vi "DOE Agilent Setup.vi"(8 "error in (no error)":errorcluster, 11 "Test Fixture Hardware":T1={"Power "={"Yokogawa"={"WT210"={"Sample Rate (1: 0.25s)"=1, "A Range (12: 20A)"=11, "V Range (6: 600V)"=4, "Power VISA Yokogawa WT210"=""}, "WT500"={"Power VISA Yokogawa WT500"="", "V Range (8: 1000V)"=6, "I Range (7: 40A)"=7, "Update Rate (3: 500ms)"=2}, "WT310_2"={"Sample Rate (1: 0.25s)"=1, "A Range (12: 20A)"=11, "V Range (6: 600V)"=4, "Power VISA Yokogawa WT310_2"=""}, "WT310_3"={"Sample Rate (1: 0.25s)"=1, "A Range (12: 20A)"=11, "V Range (6: 600V)"=4, "Power VISA Yokogawa WT310_3"=""}}, "Aplus"={"Aplus IP Address"="192.168.1.101", "Remote Port"=502, "Instrument"="APLUS", "Instr Driver Revision"="1.03.0053"}, "Power Limits"={"Crest Factor"={"Upper Limit"=1.49, "Lower Limit"=1.34}, "Harmonic Content"={"Uthd"=2.0}, "Voltage"={"% Error"=2.0}, "Stability"={"<1 Watt "={"Wattage"=1.0, "Slope (mW/H)"=10.0}, ">1 Watt"={"1%Power/Hour"=1.0}}}, "Nominal Voltage"=120, "Time Limit (s)"=10800.0, "Power Variation Limit (%)"=50.0, "Power Supply"={"Chroma 61605"="CHROMA", "Use Chroma?"=FALSE}}, "Weight Scale"={"Com Options"={"IND560Scale VISA"="MW100", "IP Address"="", "Remote Port"=502, "Setra Scale VISA"="MW100", "GSE 350"="GSE350"}, "Select Scale"=""}, "Flow Rates"={"Laurel Cold IP Address"="", "Laurel Hot IP Address"="", "Hot Water Laurel VISA"="LaurelMeter_Hot", "Cold Water Laurel VISA"="LaurelMeter_Cold", "Remote Port"=0, "Laurel Communication Type"="", "Meters To Collect (Hot Cold)"="", "HOT Laurel Reference"=refnum, "COLD Laurel Reference"=refnum, "Modbus Hot Ref"=refnum}, "Analog Data"={"Agilent"={"Agilent 34972_1"="34972A_1", "Agilent 34972_2"="34972A_2", "Agilent 34972_3"="34972A_3", "Agilent 34972_4"="34972A_3", "Agilent 34972_5"="34972A_3", "Agilent 34972_6"="34972A_3", "Agilent Gain"=0.0, "TC Type (K,J,T)"="", "Instrument IDN?"="", "TC Channels-List"="", "Analog Channels-List"="", "Agilent Cluster Array"=[], "TC Channels-List 2"="", "Analog Channels-List 2"=""}, "Yokogawa"={"MW100"="MW100", "Intellifaucet"=FALSE}, "Select Analog"="", "TC Coefficients"={"TC Coefficients 1"=[], "TC Coefficients 2"=[], "TC Coefficients 3"=[], "TC Coefficients 4"=[], "TC Coefficients 5"=[], "TC Coefficients 6"=[], "TC Coefficients 7"=[]}, "NI Tasks (Dryer DOE)"=["TC Temps-Module 1", "TC Temps-Module 2", "TC Temps-Module 3", "TC Temps-Module 4", "TC Temps-Module 5", "Gas and Temp-Module 6", "AC_DC Events-Module 7"], "Laurel Analog"={"Laurel IP (Water Temp)"="", "Laurel IP (Pressure)"=""}}, "ITHX-Temp Humidity"={"IP Address 1"="", "Remote Port"=0, "IP Address 2"="", "IP Address 3"=""}, "Gas Meter"={"Gas Meter 1"="COM3", "Gas Meter 2"="COM4", "Gas Meter 3"="COM5", "Gas Meter 4"="COM6", "Gas Meter 5"="COM7", "Gas Meter 6"="COM8", "Data Frame Format"={"Absolute Pressure"=FALSE, "Gauge/Diff. Pressure"=FALSE, "Barometric Pressure"=FALSE, "Temperature"=FALSE, "Volumetric"=FALSE, "Mass"=FALSE, "Setpoint"=FALSE, "Valve Drive"=FALSE, "Totalizer"=FALSE, "Totalizer Timer"=FALSE, "Totalizer Average Flow"=FALSE, "Totalizer Peak Flow"=FALSE, "Gas Selected"=FALSE, "Tot. Timer Format"=0}, "Measurement Data"={"Absolute Pressure"=0.0, "Gauge/Diff. Pressure"=0.0, "Barometric Pressure"=0.0, "Temperature"=0.0, "Volumetric Flow"=0.0, "Mass Flow"=0.0, "Setpoint"=0.0, "Valve Drive"=0.0, "Totalizer"=0.0, "[hr]"=0.0, "[min]"=0.0, "[sec]"=0.0, "Totalizer Average Flow"=0.0, "Totalizer Peak Flow"=0.0, "Gas selected"="COM3"}, "Measurement Units"={"Software Rev"="COM4", "Model Number"="COM5", "Manufacturer Info"="COM6", "Software Sub-Rev"="COM7", "Board Rev"="COM8", "Units of Measure Input"={"Abs. Pressure"="", "Gauge/Diff. Press."="", "Barometric Press."="", "Temperature"="", "Volume"="", "Mass"="", "Setpoint"="", "Valve Drive"="", "Totalizer"="", "Tot. Timer"="", "Tot. Avg. Flow"="", "Tot. Peak Flow"=""}}}, "Barometric Pressure"={"HEISE 901A"="HEISE", "Use Barometer?"=FALSE}, "Gas Analysis"={"Ultramat 23 VISA"="ULTRAMAT"}, "Inficon Micro GC"={"Propane IP Address"="192.168.1.33", "Natural Gas  IP Address"="192.168.1.32", "Remote Port"=502}} {"Power"."Yokogawa"."WT310_3"."V Range (6: 600V)" items=["Auto", "15V", "30V", "60V", "150V", "300V", "600V"]; "Power"."Yokogawa"."WT310_3"."A Range (12: 20A)" items=["Auto", "5mA", "10mA", "20mA", "50mA", "100mA", "200mA", "0.5A", "1A", "2A", "5A", "10A", "20A", "50mV", "100mV", "200mV", "2.5V", "5V", "10V"]; "Power"."Yokogawa"."WT310_3"."Sample Rate (1: 0.25s)" items=["0.1s", "0.25s", "0.5s", "1s", "2s", "5s"]; "Power"."Yokogawa"."WT310_2"."V Range (6: 600V)" items=["Auto", "15V", "30V", "60V", "150V", "300V", "600V"]; "Power"."Yokogawa"."WT310_2"."A Range (12: 20A)" items=["Auto", "5mA", "10mA", "20mA", "50mA", "100mA", "200mA", "0.5A", "1A", "2A", "5A", "10A", "20A", "50mV", "100mV", "200mV", "2.5V", "5V", "10V"]; "Power"."Yokogawa"."WT310_2"."Sample Rate (1: 0.25s)" items=["0.1s", "0.25s", "0.5s", "1s", "2s", "5s"]; "Power"."Yokogawa"."WT500"."Update Rate (3: 500ms)" items=["-", "100ms", "200ms", "500ms", "1s", "2s", "5s"]; "Power"."Yokogawa"."WT500"."I Range (7: 40A)" items=["AUTO", "500 mA", "1 A", "2 A", "5 A", "10 A", "20 A", "40 A", "S-AUTO", "50 mV", "100 mV", "200 mV", "500 mV", "1 V", "2 V", "5 V", "10 V", "250 mA", "500 mA", "1 A", "2.5 A", "5 A", "10 A", "20 A", "25 mV", "50 mV", "100 mV", "250 mV", "500 mV", "1 V", "2.5 V", "5 V"]; "Power"."Yokogawa"."WT500"."V Range (8: 1000V)" items=["AUTO", "15", "30", "60", "100", "150", "300", "600", "1000", "7.5", "15", "30", "50", "75", "150", "300", "500"]; "Power"."Yokogawa"."WT210"."V Range (6: 600V)" items=["Auto", "15V", "30V", "60V", "150V", "300V", "600V"]; "Power"."Yokogawa"."WT210"."A Range (12: 20A)" items=["Auto", "5mA", "10mA", "20mA", "50mA", "100mA", "200mA", "0.5A", "1A", "2A", "5A", "10A", "20A", "50mV", "100mV", "200mV", "2.5V", "5V", "10V"]; "Power"."Yokogawa"."WT210"."Sample Rate (1: 0.25s)" items=["0.1s", "0.25s", "0.5s", "1s", "2s", "5s"]}) -> (0 "error out":errorcluster, 3 "Test Fixture Hardware Output":T1={"Power "={"Yokogawa"={"WT210"={"Sample Rate (1: 0.25s)"=1, "A Range (12: 20A)"=11, "V Range (6: 600V)"=4, "Power VISA Yokogawa WT210"=""}, "WT500"={"Power VISA Yokogawa WT500"="", "V Range (8: 1000V)"=6, "I Range (7: 40A)"=7, "Update Rate (3: 500ms)"=2}, "WT310_2"={"Sample Rate (1: 0.25s)"=1, "A Range (12: 20A)"=11, "V Range (6: 600V)"=4, "Power VISA Yokogawa WT310_2"=""}, "WT310_3"={"Sample Rate (1: 0.25s)"=1, "A Range (12: 20A)"=11, "V Range (6: 600V)"=4, "Power VISA Yokogawa WT310_3"=""}}, "Aplus"={"Aplus IP Address"="192.168.1.101", "Remote Port"=502, "Instrument"="APLUS", "Instr Driver Revision"="1.03.0053"}, "Power Limits"={"Crest Factor"={"Upper Limit"=1.49, "Lower Limit"=1.34}, "Harmonic Content"={"Uthd"=2.0}, "Voltage"={"% Error"=2.0}, "Stability"={"<1 Watt "={"Wattage"=1.0, "Slope (mW/H)"=10.0}, ">1 Watt"={"1%Power/Hour"=1.0}}}, "Nominal Voltage"=120, "Time Limit (s)"=10800.0, "Power Variation Limit (%)"=50.0, "Power Supply"={"Chroma 61605"="CHROMA", "Use Chroma?"=FALSE}}, "Weight Scale"={"Com Options"={"IND560Scale VISA"="MW100", "IP Address"="", "Remote Port"=502, "Setra Scale VISA"="MW100", "GSE 350"="GSE350"}, "Select Scale"=""}, "Flow Rates"={"Laurel Cold IP Address"="", "Laurel Hot IP Address"="", "Hot Water Laurel VISA"="LaurelMeter_Hot", "Cold Water Laurel VISA"="LaurelMeter_Cold", "Remote Port"=0, "Laurel Communication Type"="", "Meters To Collect (Hot Cold)"="", "HOT Laurel Reference"=refnum, "COLD Laurel Reference"=refnum, "Modbus Hot Ref"=refnum}, "Analog Data"={"Agilent"={"Agilent 34972_1"="34972A_1", "Agilent 34972_2"="34972A_2", "Agilent 34972_3"="34972A_3", "Agilent 34972_4"="34972A_3", "Agilent 34972_5"="34972A_3", "Agilent 34972_6"="34972A_3", "Agilent Gain"=0.0, "TC Type (K,J,T)"="", "Instrument IDN?"="", "TC Channels-List"="", "Analog Channels-List"="", "Agilent Cluster Array"=[], "TC Channels-List 2"="", "Analog Channels-List 2"=""}, "Yokogawa"={"MW100"="MW100", "Intellifaucet"=FALSE}, "Select Analog"="", "TC Coefficients"={"TC Coefficients 1"=[], "TC Coefficients 2"=[], "TC Coefficients 3"=[], "TC Coefficients 4"=[], "TC Coefficients 5"=[], "TC Coefficients 6"=[], "TC Coefficients 7"=[]}, "NI Tasks (Dryer DOE)"=["TC Temps-Module 1", "TC Temps-Module 2", "TC Temps-Module 3", "TC Temps-Module 4", "TC Temps-Module 5", "Gas and Temp-Module 6", "AC_DC Events-Module 7"], "Laurel Analog"={"Laurel IP (Water Temp)"="", "Laurel IP (Pressure)"=""}}, "ITHX-Temp Humidity"={"IP Address 1"="", "Remote Port"=0, "IP Address 2"="", "IP Address 3"=""}, "Gas Meter"={"Gas Meter 1"="COM3", "Gas Meter 2"="COM4", "Gas Meter 3"="COM5", "Gas Meter 4"="COM6", "Gas Meter 5"="COM7", "Gas Meter 6"="COM8", "Data Frame Format"={"Absolute Pressure"=FALSE, "Gauge/Diff. Pressure"=FALSE, "Barometric Pressure"=FALSE, "Temperature"=FALSE, "Volumetric"=FALSE, "Mass"=FALSE, "Setpoint"=FALSE, "Valve Drive"=FALSE, "Totalizer"=FALSE, "Totalizer Timer"=FALSE, "Totalizer Average Flow"=FALSE, "Totalizer Peak Flow"=FALSE, "Gas Selected"=FALSE, "Tot. Timer Format"=0}, "Measurement Data"={"Absolute Pressure"=0.0, "Gauge/Diff. Pressure"=0.0, "Barometric Pressure"=0.0, "Temperature"=0.0, "Volumetric Flow"=0.0, "Mass Flow"=0.0, "Setpoint"=0.0, "Valve Drive"=0.0, "Totalizer"=0.0, "[hr]"=0.0, "[min]"=0.0, "[sec]"=0.0, "Totalizer Average Flow"=0.0, "Totalizer Peak Flow"=0.0, "Gas selected"="COM3"}, "Measurement Units"={"Software Rev"="COM4", "Model Number"="COM5", "Manufacturer Info"="COM6", "Software Sub-Rev"="COM7", "Board Rev"="COM8", "Units of Measure Input"={"Abs. Pressure"="", "Gauge/Diff. Press."="", "Barometric Press."="", "Temperature"="", "Volume"="", "Mass"="", "Setpoint"="", "Valve Drive"="", "Totalizer"="", "Tot. Timer"="", "Tot. Avg. Flow"="", "Tot. Peak Flow"=""}}}, "Barometric Pressure"={"HEISE 901A"="HEISE", "Use Barometer?"=FALSE}, "Gas Analysis"={"Ultramat 23 VISA"="ULTRAMAT"}, "Inficon Micro GC"={"Propane IP Address"="192.168.1.33", "Natural Gas  IP Address"="192.168.1.32", "Remote Port"=502}} {"Power"."Yokogawa"."WT310_3"."V Range (6: 600V)" items=["Auto", "15V", "30V", "60V", "150V", "300V", "600V"]; "Power"."Yokogawa"."WT310_3"."A Range (12: 20A)" items=["Auto", "5mA", "10mA", "20mA", "50mA", "100mA", "200mA", "0.5A", "1A", "2A", "5A", "10A", "20A", "50mV", "100mV", "200mV", "2.5V", "5V", "10V"]; "Power"."Yokogawa"."WT310_3"."Sample Rate (1: 0.25s)" items=["0.1s", "0.25s", "0.5s", "1s", "2s", "5s"]; "Power"."Yokogawa"."WT310_2"."V Range (6: 600V)" items=["Auto", "15V", "30V", "60V", "150V", "300V", "600V"]; "Power"."Yokogawa"."WT310_2"."A Range (12: 20A)" items=["Auto", "5mA", "10mA", "20mA", "50mA", "100mA", "200mA", "0.5A", "1A", "2A", "5A", "10A", "20A", "50mV", "100mV", "200mV", "2.5V", "5V", "10V"]; "Power"."Yokogawa"."WT310_2"."Sample Rate (1: 0.25s)" items=["0.1s", "0.25s", "0.5s", "1s", "2s", "5s"]; "Power"."Yokogawa"."WT500"."Update Rate (3: 500ms)" items=["-", "100ms", "200ms", "500ms", "1s", "2s", "5s"]; "Power"."Yokogawa"."WT500"."I Range (7: 40A)" items=["AUTO", "500 mA", "1 A", "2 A", "5 A", "10 A", "20 A", "40 A", "S-AUTO", "50 mV", "100 mV", "200 mV", "500 mV", "1 V", "2 V", "5 V", "10 V", "250 mA", "500 mA", "1 A", "2.5 A", "5 A", "10 A", "20 A", "25 mV", "50 mV", "100 mV", "250 mV", "500 mV", "1 V", "2.5 V", "5 V"]; "Power"."Yokogawa"."WT500"."V Range (8: 1000V)" items=["AUTO", "15", "30", "60", "100", "150", "300", "600", "1000", "7.5", "15", "30", "50", "75", "150", "300", "500"]; "Power"."Yokogawa"."WT210"."V Range (6: 600V)" items=["Auto", "15V", "30V", "60V", "150V", "300V", "600V"]; "Power"."Yokogawa"."WT210"."A Range (12: 20A)" items=["Auto", "5mA", "10mA", "20mA", "50mA", "100mA", "200mA", "0.5A", "1A", "2A", "5A", "10A", "20A", "50mV", "100mV", "200mV", "2.5V", "5V", "10V"]; "Power"."Yokogawa"."WT210"."Sample Rate (1: 0.25s)" items=["0.1s", "0.25s", "0.5s", "1s", "2s", "5s"]})   [LabVIEW 2020]
uses:
  Type Definitions/DOE Test Fixture Hardware.ctl
  <vilib>/NI/Modbus Library/API/Master/Modbus Master.lvclass
  Utility/Type Definitions/UTILITY Power Inputs Control.ctl
  Drivers/IND560 Scale Monitor/Type Definitions/IND560 Configuration.ctl
  Hybrid Water Heater/Type Definitions/HEWH Agilent Cluster.ctl
  Utility/Type Definitions/UTILITY TC Coefficients.ctl
  Drivers/Omega FMA-1600A Series Gas Flow Meter/Type Definitions/FMA1600A COM Ports.ctl
  Drivers/Alicat Gas Meter Driver/Sub-VIs/Data Frame.ctl
  Drivers/Alicat Gas Meter Driver/Sub-VIs/Data Cluster.ctl
  Drivers/Omega FMA-1600A Series Gas Flow Meter/Type Definitions/FMA1600A Units String.ctl
  Drivers/Alicat Gas Meter Driver/Sub-VIs/Units of Measure.ctl
  <vilib>/Utility/error.llb/whitespace.ctl
  Drivers/Agilent 34972/Agilent 34970.lvlib
panel:
  # "Totalizer Timer"
  # "Totalizer Timer"
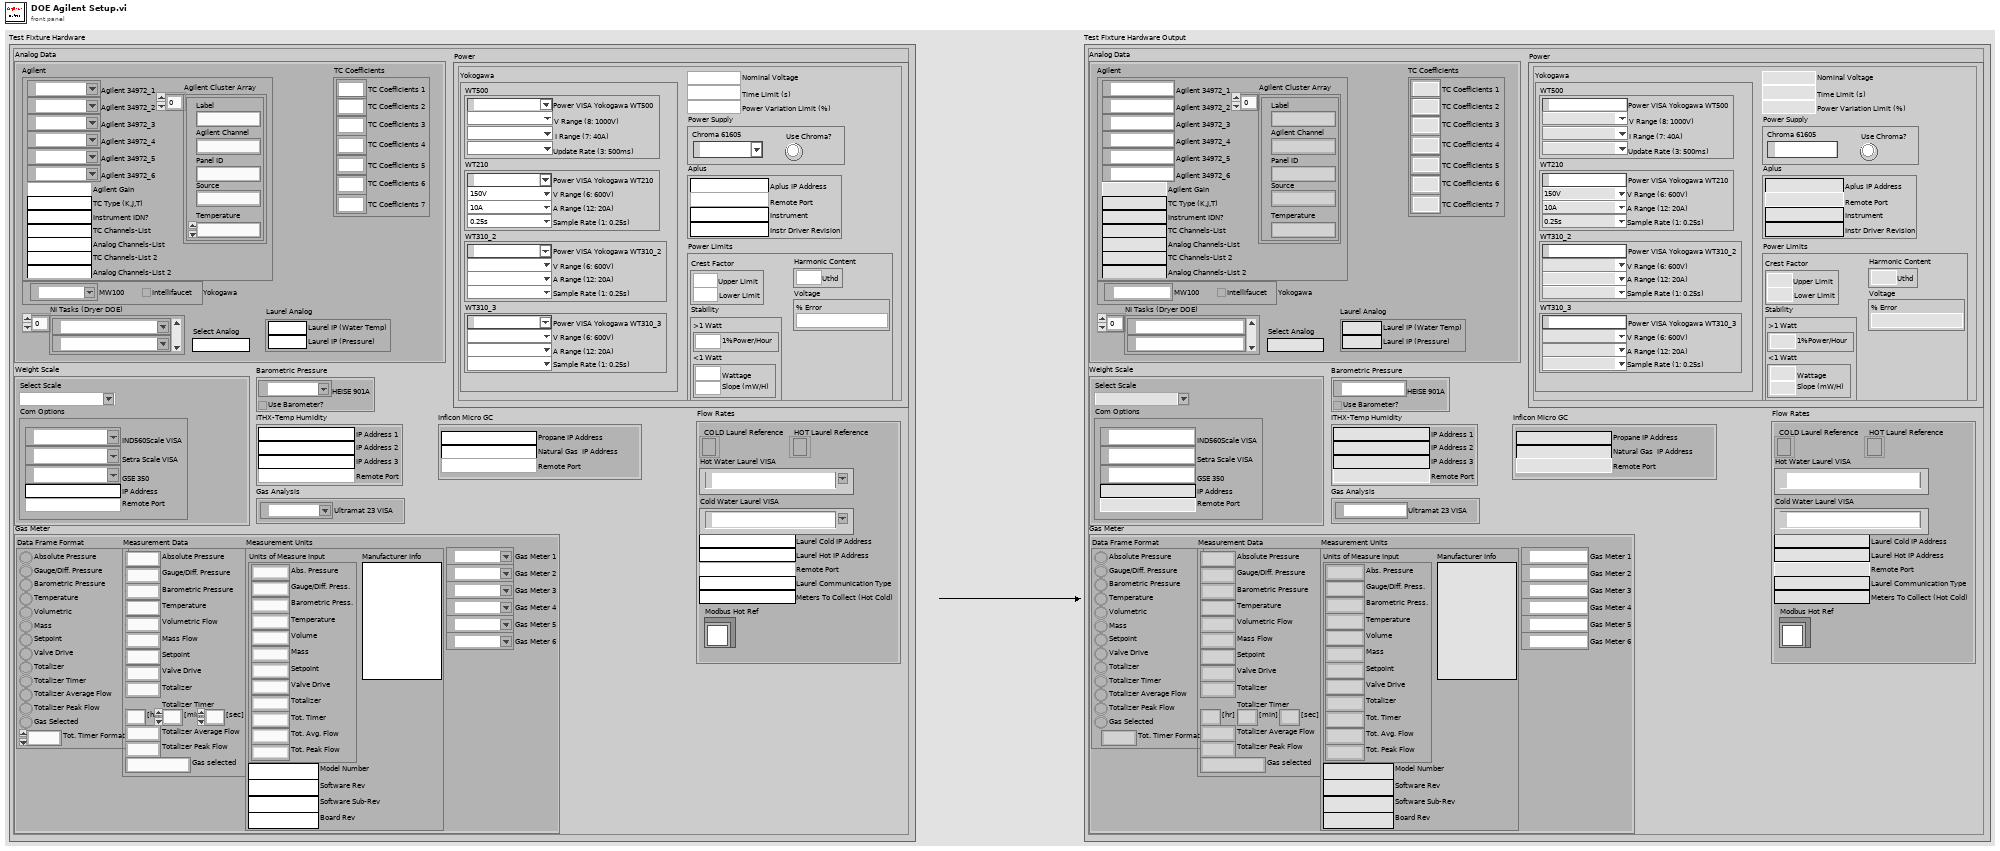
[diagram p1: front panel]
types:
  T1 = typedef "DOE Test Fixture Hardware.ctl" = cluster{"Power ":T2, "Weight Scale":cluster{"Com Options":T3, "Select Scale":string}, "Flow Rates":cluster{"Laurel Cold IP Address":string, "Laurel Hot IP Address":string, "Hot Water Laurel VISA":refnum<visa-resource-name>, "Cold Water Laurel VISA":refnum<visa-resource-name>, "Remote Port":u16, "Laurel Communication Type":string, "Meters To Collect (Hot Cold)":string, "HOT Laurel Reference":refnum<k5>, "COLD Laurel Reference":refnum<k5>, "Modbus Hot Ref":refnum<class "Modbus Master.lvclass">}, "Analog Data":cluster{"Agilent":cluster{"Agilent 34972_1":refnum<visa-resource-name>, "Agilent 34972_2":refnum<visa-resource-name>, "Agilent 34972_3":refnum<visa-resource-name>, "Agilent 34972_4":refnum<visa-resource-name>, "Agilent 34972_5":refnum<visa-resource-name>, "Agilent 34972_6":refnum<visa-resource-name>, "Agilent Gain":dbl, "TC Type (K,J,T)":string, "Instrument IDN?":string, "TC Channels-List":string, "Analog Channels-List":string, "Agilent Cluster Array":T4[], "TC Channels-List 2":string, "Analog Channels-List 2":string}, "Yokogawa":cluster{"MW100":refnum<visa-resource-name>, "Intellifaucet":bool}, "Select Analog":string, "TC Coefficients":T5, "NI Tasks (Dryer DOE)":refnum<k21>[], "Laurel Analog":cluster{"Laurel IP (Water Temp)":string, "Laurel IP (Pressure)":string}}, "ITHX-Temp Humidity":cluster{"IP Address 1":string, "Remote Port":u16, "IP Address 2":string, "IP Address 3":string}, "Gas Meter":T6, "Barometric Pressure":cluster{"HEISE 901A":refnum<visa-resource-name>, "Use Barometer?":bool}, "Gas Analysis":cluster{"Ultramat 23 VISA":refnum<visa-resource-name>}, "Inficon Micro GC":cluster{"Propane IP Address":string, "Natural Gas  IP Address":string, "Remote Port":u16}}
  T2 = typedef "UTILITY Power Inputs Control.ctl" = cluster{"Yokogawa":cluster{"WT210":cluster{"Sample Rate (1: 0.25s)":i32, "A Range (12: 20A)":i32, "V Range (6: 600V)":i32, "Power VISA Yokogawa WT210":refnum<visa-resource-name>}, "WT500":cluster{"Power VISA Yokogawa WT500":refnum<visa-resource-name>, "V Range (8: 1000V)":i32, "I Range (7: 40A)":i32, "Update Rate (3: 500ms)":i32}, "WT310_2":cluster{"Sample Rate (1: 0.25s)":i32, "A Range (12: 20A)":i32, "V Range (6: 600V)":i32, "Power VISA Yokogawa WT310_2":refnum<visa-resource-name>}, "WT310_3":cluster{"Sample Rate (1: 0.25s)":i32, "A Range (12: 20A)":i32, "V Range (6: 600V)":i32, "Power VISA Yokogawa WT310_3":refnum<visa-resource-name>}}, "Aplus":cluster{"Aplus IP Address":string, "Remote Port":i32, "Instrument":string, "Instr Driver Revision":string}, "Power Limits":cluster{"Crest Factor":cluster{"Upper Limit":dbl, "Lower Limit":dbl}, "Harmonic Content":cluster{"Uthd":dbl}, "Voltage":cluster{"% Error":dbl}, "Stability":cluster{"<1 Watt ":cluster{"Wattage":dbl, "Slope (mW/H)":dbl}, ">1 Watt":cluster{"1%Power/Hour":dbl}}}, "Nominal Voltage":i32, "Time Limit (s)":dbl, "Power Variation Limit (%)":dbl, "Power Supply":cluster{"Chroma 61605":refnum<visa-resource-name>, "Use Chroma?":bool}}
  T3 = typedef "IND560 Configuration.ctl" = cluster{"IND560Scale VISA":refnum<visa-resource-name>, "IP Address":string, "Remote Port":u16, "Setra Scale VISA":refnum<visa-resource-name>, "GSE 350":refnum<visa-resource-name>}
  T4 = typedef "HEWH Agilent Cluster.ctl" = cluster{"Label":string, "Agilent Channel":string, "Panel ID":string, "Source":string, "Temperature":dbl}
  T5 = typedef "UTILITY TC Coefficients.ctl" = cluster{"TC Coefficients 1":dbl[], "TC Coefficients 2":dbl[], "TC Coefficients 3":dbl[], "TC Coefficients 4":dbl[], "TC Coefficients 5":dbl[], "TC Coefficients 6":dbl[], "TC Coefficients 7":dbl[]}
  T6 = typedef "FMA1600A COM Ports.ctl" = cluster{"Gas Meter 1":refnum<visa-resource-name>, "Gas Meter 2":refnum<visa-resource-name>, "Gas Meter 3":refnum<visa-resource-name>, "Gas Meter 4":refnum<visa-resource-name>, "Gas Meter 5":refnum<visa-resource-name>, "Gas Meter 6":refnum<visa-resource-name>, "Data Frame Format":T7, "Measurement Data":T8, "Measurement Units":T9}
  T7 = typedef "Data Frame.ctl" = cluster{"Absolute Pressure":bool, "Gauge/Diff. Pressure":bool, "Barometric Pressure":bool, "Temperature":bool, "Volumetric":bool, "Mass":bool, "Setpoint":bool, "Valve Drive":bool, "Totalizer":bool, "Totalizer Timer":bool, "Totalizer Average Flow":bool, "Totalizer Peak Flow":bool, "Gas Selected":bool, "Tot. Timer Format":u16}
  T8 = typedef "Data Cluster.ctl" = cluster{"Absolute Pressure":dbl, "Gauge/Diff. Pressure":dbl, "Barometric Pressure":dbl, "Temperature":dbl, "Volumetric Flow":dbl, "Mass Flow":dbl, "Setpoint":dbl, "Valve Drive":dbl, "Totalizer":dbl, "[hr]":dbl, "[min]":dbl, "[sec]":dbl, "Totalizer Average Flow":dbl, "Totalizer Peak Flow":dbl, "Gas selected":string}
  T9 = typedef "FMA1600A Units String.ctl" = cluster{"Software Rev":string, "Model Number":string, "Manufacturer Info":string, "Software Sub-Rev":string, "Board Rev":string, "Units of Measure Input":T10}
  T10 = typedef "Units of Measure.ctl" = cluster{"Abs. Pressure":string, "Gauge/Diff. Press.":string, "Barometric Press.":string, "Temperature":string, "Volume":string, "Mass":string, "Setpoint":string, "Valve Drive":string, "Totalizer":string, "Tot. Timer":string, "Tot. Avg. Flow":string, "Tot. Peak Flow":string}
  T11 = typedef "whitespace.ctl" = u16
  T12 = enum16{"Temperature", "DC Voltage", "AC Voltage", "DC Current", "AC Current", "Resistance", "4-Wire Resistance", "Frequency", "Period", "Digital", "Totalizer"}
  T13 = cluster{"Timeout Value (10000)":u32, "Baud Rate (57600)":enum16{"1200", "2400", "4800", "9600", "19200", "38400", "57600", "115200"}, "Flow Control (1:XON/XOFF)":enum16{"None", "XON / XOFF", "RTS / CTS", "DTR / DSR"}}
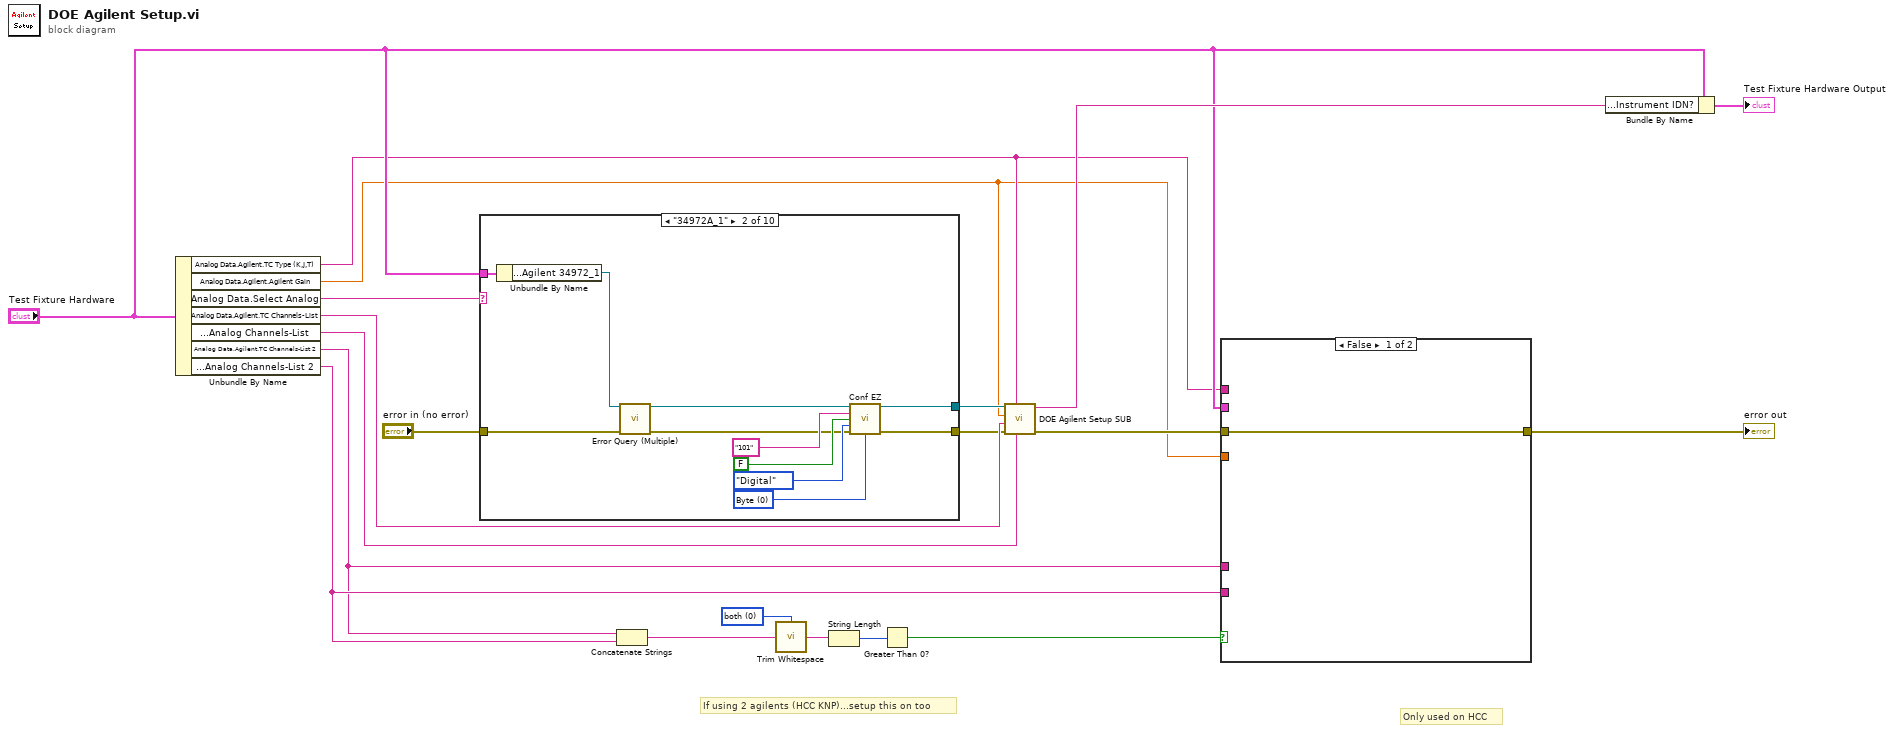
[diagram p0: block diagram]
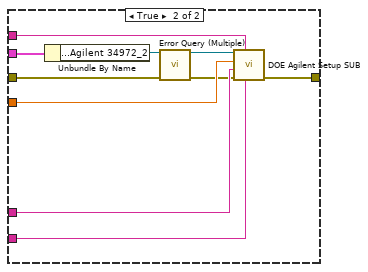
[diagram p2: hidden frame]
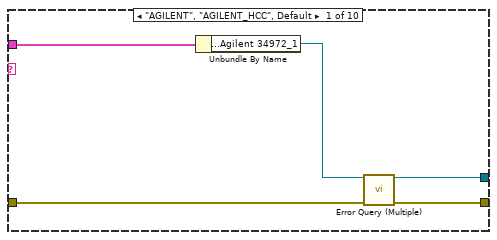
[diagram p3: hidden frame]
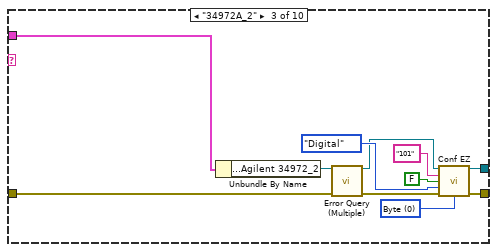
[diagram p4: hidden frame]
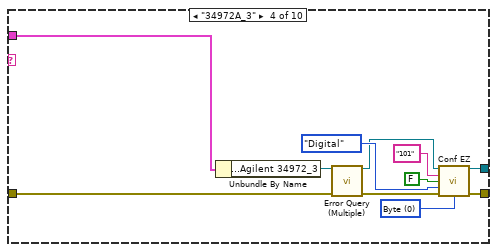
[diagram p5: hidden frame]
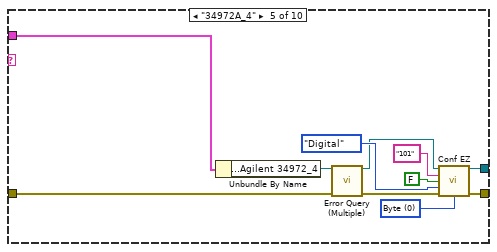
[diagram p6: hidden frame]
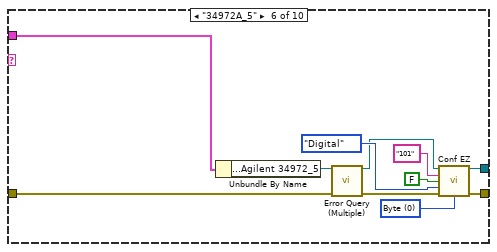
[diagram p7: hidden frame]
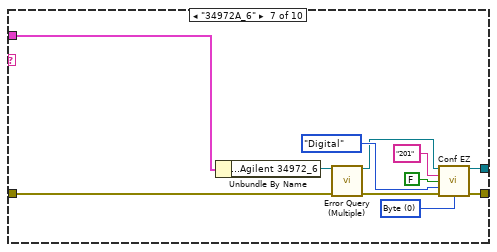
[diagram p8: hidden frame]
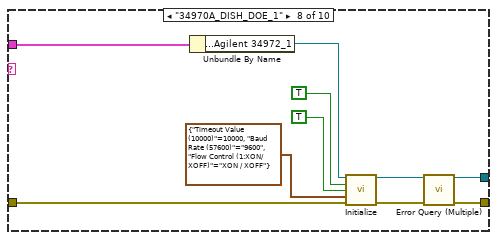
[diagram p9: hidden frame]
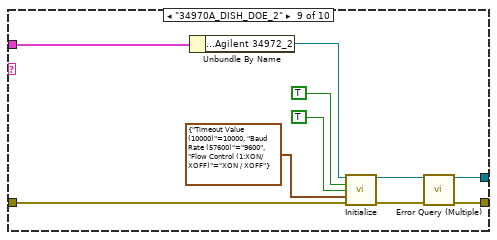
[diagram p10: hidden frame]
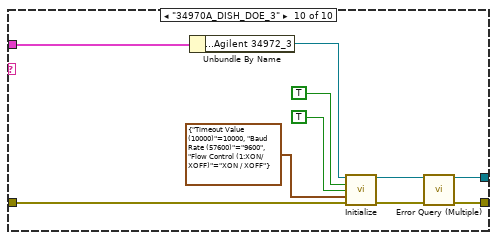
[diagram p11: hidden frame]
diagram:
  w11 = T11 0 items=["both", "start of string", "end of string"] ("location (both)")
  # "Only used on HCC"
  # "If using 2 agilents (HCC KNP)...setup this on too"
  n1 = Unbundle By Name("Test Fixture Hardware") -> ("Analog Data.Agilent.TC Type (K,J,T)"=w2:string, "Analog Data.Agilent.Agilent Gain"=w1:dbl, "Analog Data.Select Analog"=w15:string, "Analog Data.Agilent.TC Channels-List"=w20:string, "Analog Data.Agilent.Analog Channels-List"=w19:string, "Analog Data.Agilent.TC Channels-List 2"=w6:string, "Analog Data.Agilent.Analog Channels-List 2"=w7:string)
  n2 = case shown="\"34972A_1\"" w15 {
    tunnel: [w22 w31 w42 w53 w64 w75 w86 w99 w109 w119] -> w16
    tunnel: "Test Fixture Hardware" -> [w25 w36 w47 w58 w69 w80 w91 w101 w111 w121]
    tunnel: "error in (no error)" -> [w24 w29 w40 w51 w62 w73 w84 w96 w106 w116]
    tunnel: [w21 w30 w41 w52 w63 w74 w85 w100 w110 w120] -> w3
    frame "AGILENT", "AGILENT_HCC", Default {
      n3 = Unbundle By Name(w25) -> ("Analog Data.Agilent.Agilent 34972_1"=w23:refnum<visa-resource-name>)
      n4 = call "Error Query (Multiple).vi"("VISA Resource Name"=w23, "error in (no error)"=w24) -> ("VISA Resource Name Out"=w22:refnum<visa-resource-name>, "error out"=w21:errorcluster)  [unwired: 10 in, 2 out]
    }
    frame "34972A_1" {
      w34 = u16 0 items=["Byte"] ("Digital (0:Byte)")
      n5 = Unbundle By Name(w36) -> ("Analog Data.Agilent.Agilent 34972_1"=w27:refnum<visa-resource-name>)
      n6 = call "Error Query (Multiple).vi"("VISA Resource Name"=w27, "error in (no error)"=w29) -> ("VISA Resource Name Out"=w26:refnum<visa-resource-name>, "error out"=w28:errorcluster)  [unwired: 10 in, 2 out]
      n7 = call "Conf EZ.vi"("VISA Resource Name"=w26, "Channel List(empty)"="101", "Set/Check (F:Set)"=FALSE, "Measurement (1:DC Volt)"=T12."Digital", "error in (no error)"=w28, "Digital (0:Byte)"=w34) -> ("VISA Resource Name Out"=w31:refnum<visa-resource-name>, "error out"=w30:errorcluster)  [unwired: 7 in, 1 out]
    }
    frame "34972A_2" {
      w45 = u16 0 items=["Byte"] ("Digital (0:Byte)")
      n8 = Unbundle By Name(w47) -> ("Analog Data.Agilent.Agilent 34972_2"=w38:refnum<visa-resource-name>)
      n9 = call "Error Query (Multiple).vi"("VISA Resource Name"=w38, "error in (no error)"=w40) -> ("VISA Resource Name Out"=w37:refnum<visa-resource-name>, "error out"=w39:errorcluster)  [unwired: 10 in, 2 out]
      n10 = call "Conf EZ.vi"("VISA Resource Name"=w37, "Channel List(empty)"="101", "Set/Check (F:Set)"=FALSE, "Measurement (1:DC Volt)"=T12."Digital", "error in (no error)"=w39, "Digital (0:Byte)"=w45) -> ("VISA Resource Name Out"=w42:refnum<visa-resource-name>, "error out"=w41:errorcluster)  [unwired: 7 in, 1 out]
    }
    frame "34972A_3" {
      w56 = u16 0 items=["Byte"] ("Digital (0:Byte)")
      n11 = Unbundle By Name(w58) -> ("Analog Data.Agilent.Agilent 34972_3"=w49:refnum<visa-resource-name>)
      n12 = call "Error Query (Multiple).vi"("VISA Resource Name"=w49, "error in (no error)"=w51) -> ("VISA Resource Name Out"=w48:refnum<visa-resource-name>, "error out"=w50:errorcluster)  [unwired: 10 in, 2 out]
      n13 = call "Conf EZ.vi"("VISA Resource Name"=w48, "Channel List(empty)"="101", "Set/Check (F:Set)"=FALSE, "Measurement (1:DC Volt)"=T12."Digital", "error in (no error)"=w50, "Digital (0:Byte)"=w56) -> ("VISA Resource Name Out"=w53:refnum<visa-resource-name>, "error out"=w52:errorcluster)  [unwired: 7 in, 1 out]
    }
    frame "34972A_4" {
      w67 = u16 0 items=["Byte"] ("Digital (0:Byte)")
      n14 = Unbundle By Name(w69) -> ("Analog Data.Agilent.Agilent 34972_4"=w60:refnum<visa-resource-name>)
      n15 = call "Error Query (Multiple).vi"("VISA Resource Name"=w60, "error in (no error)"=w62) -> ("VISA Resource Name Out"=w59:refnum<visa-resource-name>, "error out"=w61:errorcluster)  [unwired: 10 in, 2 out]
      n16 = call "Conf EZ.vi"("VISA Resource Name"=w59, "Channel List(empty)"="101", "Set/Check (F:Set)"=FALSE, "Measurement (1:DC Volt)"=T12."Digital", "error in (no error)"=w61, "Digital (0:Byte)"=w67) -> ("VISA Resource Name Out"=w64:refnum<visa-resource-name>, "error out"=w63:errorcluster)  [unwired: 7 in, 1 out]
    }
    frame "34972A_5" {
      w78 = u16 0 items=["Byte"] ("Digital (0:Byte)")
      n17 = Unbundle By Name(w80) -> ("Analog Data.Agilent.Agilent 34972_5"=w71:refnum<visa-resource-name>)
      n18 = call "Error Query (Multiple).vi"("VISA Resource Name"=w71, "error in (no error)"=w73) -> ("VISA Resource Name Out"=w70:refnum<visa-resource-name>, "error out"=w72:errorcluster)  [unwired: 10 in, 2 out]
      n19 = call "Conf EZ.vi"("VISA Resource Name"=w70, "Channel List(empty)"="101", "Set/Check (F:Set)"=FALSE, "Measurement (1:DC Volt)"=T12."Digital", "error in (no error)"=w72, "Digital (0:Byte)"=w78) -> ("VISA Resource Name Out"=w75:refnum<visa-resource-name>, "error out"=w74:errorcluster)  [unwired: 7 in, 1 out]
    }
    frame "34972A_6" {
      w89 = u16 0 items=["Byte"] ("Digital (0:Byte)")
      n20 = Unbundle By Name(w91) -> ("Analog Data.Agilent.Agilent 34972_6"=w82:refnum<visa-resource-name>)
      n21 = call "Error Query (Multiple).vi"("VISA Resource Name"=w82, "error in (no error)"=w84) -> ("VISA Resource Name Out"=w81:refnum<visa-resource-name>, "error out"=w83:errorcluster)  [unwired: 10 in, 2 out]
      n22 = call "Conf EZ.vi"("VISA Resource Name"=w81, "Channel List(empty)"="201", "Set/Check (F:Set)"=FALSE, "Measurement (1:DC Volt)"=T12."Digital", "error in (no error)"=w83, "Digital (0:Byte)"=w89) -> ("VISA Resource Name Out"=w86:refnum<visa-resource-name>, "error out"=w85:errorcluster)  [unwired: 7 in, 1 out]
    }
    frame "34970A_DISH_DOE_1" {
      n23 = Unbundle By Name(w101) -> ("Analog Data.Agilent.Agilent 34972_1"=w98:refnum<visa-resource-name>)
      n24 = call "Initialize.vi"("VISA Resource Name"=w98, "ID Query (T: Check)"=TRUE, "Reset (T: Reset)"=TRUE, "Serial Port Configuration"=T13 {"Timeout Value (10000)"=10000, "Baud Rate (57600)"=enum."9600", "Flow Control (1:XON/XOFF)"=enum."XON / XOFF"}, "error in (no error)"=w96) -> ("VISA Resource Name Out"=w97:refnum<visa-resource-name>, "error out"=w95:errorcluster)  [unwired: 9 in]
      n25 = call "Error Query (Multiple).vi"("VISA Resource Name"=w97, "error in (no error)"=w95) -> ("VISA Resource Name Out"=w99:refnum<visa-resource-name>, "error out"=w100:errorcluster)  [unwired: 10 in, 2 out]
    }
    frame "34970A_DISH_DOE_2" {
      n26 = Unbundle By Name(w111) -> ("Analog Data.Agilent.Agilent 34972_2"=w108:refnum<visa-resource-name>)
      n27 = call "Initialize.vi"("VISA Resource Name"=w108, "ID Query (T: Check)"=TRUE, "Reset (T: Reset)"=TRUE, "Serial Port Configuration"=T13 {"Timeout Value (10000)"=10000, "Baud Rate (57600)"=enum."9600", "Flow Control (1:XON/XOFF)"=enum."XON / XOFF"}, "error in (no error)"=w106) -> ("VISA Resource Name Out"=w107:refnum<visa-resource-name>, "error out"=w105:errorcluster)  [unwired: 9 in]
      n28 = call "Error Query (Multiple).vi"("VISA Resource Name"=w107, "error in (no error)"=w105) -> ("VISA Resource Name Out"=w109:refnum<visa-resource-name>, "error out"=w110:errorcluster)  [unwired: 10 in, 2 out]
    }
    frame "34970A_DISH_DOE_3" {
      n29 = Unbundle By Name(w121) -> ("Analog Data.Agilent.Agilent 34972_3"=w118:refnum<visa-resource-name>)
      n30 = call "Initialize.vi"("VISA Resource Name"=w118, "ID Query (T: Check)"=TRUE, "Reset (T: Reset)"=TRUE, "Serial Port Configuration"=T13 {"Timeout Value (10000)"=10000, "Baud Rate (57600)"=enum."9600", "Flow Control (1:XON/XOFF)"=enum."XON / XOFF"}, "error in (no error)"=w116) -> ("VISA Resource Name Out"=w117:refnum<visa-resource-name>, "error out"=w115:errorcluster)  [unwired: 9 in]
      n31 = call "Error Query (Multiple).vi"("VISA Resource Name"=w117, "error in (no error)"=w115) -> ("VISA Resource Name Out"=w119:refnum<visa-resource-name>, "error out"=w120:errorcluster)  [unwired: 10 in, 2 out]
    }
  }
  n32 = Concatenate Strings(w6, w7) -> (w12:string)
  n33 = call <vilib>:"Trim Whitespace.vi"("string"=w12, "location (both)"=w11) -> ("trimmed string"=w10:string)
  n34 = String Length(string=w10) -> (length=w9:i32)
  n35 = Greater Than 0?(x=w9) -> (x > 0?=w8:bool)
  n36 = call "DOE Agilent Setup SUB.vi"("Analog Channels-List"=w19, "TC Type (K,J,T)"=w2, "error in (no error)"=w3, "TC Channels-List"=w20, "Agilent Gain"=w1, "VISA Refnum in"=w16) -> ("error out"=w14:errorcluster, "Instrument IDN"=w18:string)  [unwired: 3 in, 1 out]
  n37 = case shown="False" w8 {
    tunnel: w14 -> [w122 w125]
    tunnel: [w122 w132] -> w13
    tunnel: w7 -> [_ w131]
    tunnel: w6 -> [_ w130]
    tunnel: w1 -> [_ w129]
    tunnel: "Test Fixture Hardware" -> [_ w128]
    tunnel: w2 -> [_ w127]
    frame False {
    }
    frame True {
      n38 = Unbundle By Name(w128) -> ("Analog Data.Agilent.Agilent 34972_2"=w126:refnum<visa-resource-name>)
      n39 = call "Error Query (Multiple).vi"("VISA Resource Name"=w126, "error in (no error)"=w125) -> ("VISA Resource Name Out"=w123:refnum<visa-resource-name>, "error out"=w124:errorcluster)  [unwired: 10 in, 2 out]
      n40 = call "DOE Agilent Setup SUB.vi"("Analog Channels-List"=w131, "TC Type (K,J,T)"=w127, "error in (no error)"=w124, "TC Channels-List"=w130, "Agilent Gain"=w129, "VISA Refnum in"=w123) -> ("error out"=w132:errorcluster)  [unwired: 3 in, 2 out]
    }
  }
  "error out" <- w13
  n41 = Bundle By Name(cluster="Test Fixture Hardware", "Analog Data.Agilent.Instrument IDN?"=w18) -> (→"Test Fixture Hardware Output":T1)
